vi "Force Stop Program wrapper.vi"(8 "error in (no error)":errorcluster caption="错误输入（无错误）", 9 "dwCANID":u32, 10 "pGWSearchPara":cluster{"dwComIndex":u32, "dwBtr":u32}, 11 "dwDevType":u32) -> (0 "error out":errorcluster caption="错误输出", 2 "pGWSearchPara out":cluster{"dwComIndex":u32, "dwBtr":u32}, 3 "function return":u32)   [LabVIEW 2016, in "UISimCanFunc_wrapper.lvlib"]
doc: "_declspec (dllexport) DWORD ForceStopProgram_wrapper(DWORD dwDevType, P_GW_SEARCH_PARA pGWSearchPara, DWORD dwCANID);"
uses:
  <userlib>/UISimCanFunc_wrapper/UISimCanFunc_wrapper.lvlib
  <userlib>/UISimCanFunc_wrapper/UISimCanFunc_wrapper.dll
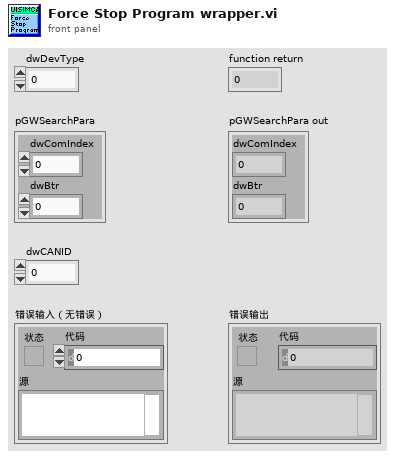
[diagram p1: front panel]
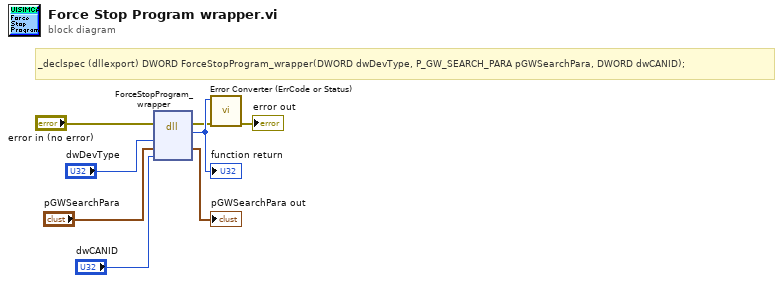
[diagram p0: block diagram]
diagram:
  # "_declspec (dllexport) DWORD ForceStopProgram_wrapper(DWORD dwDevType, P_GW_SEARCH_PARA pGWSearchPara, DWORD dwCANID);"
  n1 = dll-call lib="C:/Program Files (x86)/National Instruments/LabVIEW 2016/user.lib/UISimCanFunc_wrapper/UISimCanFunc_wrapper.*" fn="ForceStopProgram_wrapper"(error in="error in (no error)", "dwDevType"="dwDevType", "pGWSearchPara"="pGWSearchPara", "dwCANID"="dwCANID") -> (error out=w2:errorcluster, w8:u32, "pGWSearchPara"=→"pGWSearchPara out":cluster{"dwComIndex":u32, "dwBtr":u32})  [unwired: 4 in, 1 out]
  "function return" <- w8
  n2 = call <userlib>:"Error Converter (ErrCode or Status).vi"("error in (no error)"=w2, "error code"=w8) -> ("error out"=→"error out":errorcluster)  [unwired: 9 in]
